vi "Pcre2GetRealMatchDataBytes8.vi"(8 "error in":errorcluster, 11 "pMatchData":u64 format="%.0x") -> (0 "error out":errorcluster, 2 "MatchDataBytes":u8[](array[numeric]) format="%02x", 3 "pMatchData":u64 format="%.0x")   [LabVIEW 2021, in "libpcre2-8.lvlib"]
uses:
  libpcre2-8.lvlib
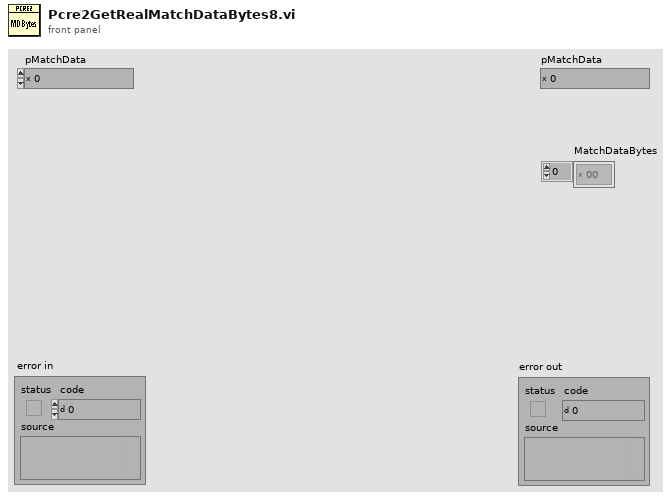
[diagram p1: front panel]
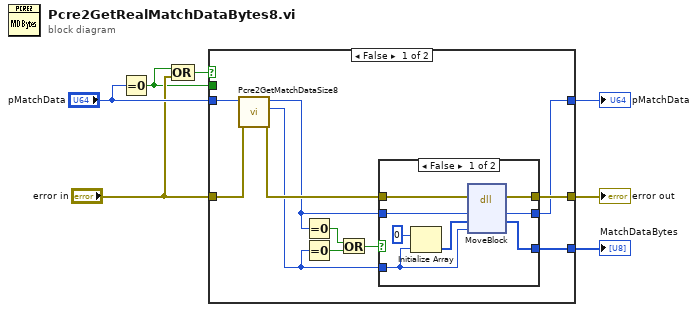
[diagram p0: block diagram]
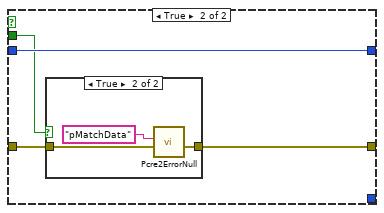
[diagram p3: hidden frame]
diagram:
  n1 = Equal To 0?(x="pMatchData") -> (x = 0?=w2:bool)
  n2 = Compound Arithmetic op=OR(w2, "error in") -> (w4:bool)
  n3 = case shown="False" w4 {
    tunnel: "error in" -> [w14 w29]
    tunnel: [w12 w31] -> w7
    tunnel: "pMatchData" -> [w18 w32]
    tunnel: [w9 w32] -> w6
    tunnel: [w11 _] -> w1
    tunnel: w2 -> [_ w30]
    frame False {
      n4 = call "Pcre2GetMatchDataSize8.vi"("error in"=w14, "pMatchData"=w18) -> ("error out"=w15:errorcluster, "MatchDataSize"=w13:u64, "pMatchData"=w10:u64)  [unwired: 7 in]
      n5 = Equal To 0?(x=w10) -> (x = 0?=w8:bool)
      n6 = Equal To 0?(x=w13) -> (x = 0?=w16:bool)
      n7 = Or(x=w8, y=w16) -> (x .or. y?=w17:bool)
      n8 = case shown="False" w17 {
        tunnel: [w25 w28] -> w9
        tunnel: [w24 _] -> w11
        tunnel: w10 -> [w26 w28]
        tunnel: w13 -> [w20 _]
        tunnel: [w23 w27] -> w12
        tunnel: w15 -> [w22 w27]
        frame False {
          n9 = Initialize Array(u8 0 ("U8"), w20) -> (w21:u8[])
          n10 = dll-call lib="LabVIEW" fn="MoveBlock"(error in=w22, "pointerSrc"=w26, "pointerDest"=w21, "size"=w20) -> (error out=w23:errorcluster, "pointerSrc"=w25:u64, "pointerDest"=w24:u8[])  [unwired: 4 in, 1 out]
        }
        frame True {
        }
      }
    }
    frame True {
      n11 = case shown="True" w30 {
        tunnel: w29 -> [w33 w35]
        tunnel: [w33 w34] -> w31
        frame False {
        }
        frame True {
          n12 = call "Pcre2ErrorNull.vi"("error in"=w35, "What"="pMatchData") -> ("error out"=w34:errorcluster)  [unwired: 9 in]
        }
      }
    }
  }
  "pMatchData" <- w6
  "error out" <- w7
  "MatchDataBytes" <- w1
